vi "Scan_ProFile_CSV_integral.vi"(5 "ProFile Path":path, 7 "Step Size in mm":sgl, 8 "Y-Axis":sgl, 9 "X-Axis":sgl, 10 "Offset Y-Axis":sgl, 11 "Offset X-Axis":sgl) -> ()   [LabVIEW 2016]
uses:
  Utility/Global Constants.vi
panel:
  out "Current Y-Step":i32
  out "Current X-Step":i32
  out "Status?":bool
  out "Abort in Progress":bool
  out "RS":bool
  in  "Abort!":bool
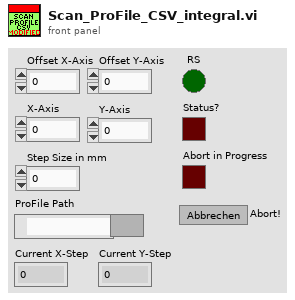
[diagram p1: front panel]
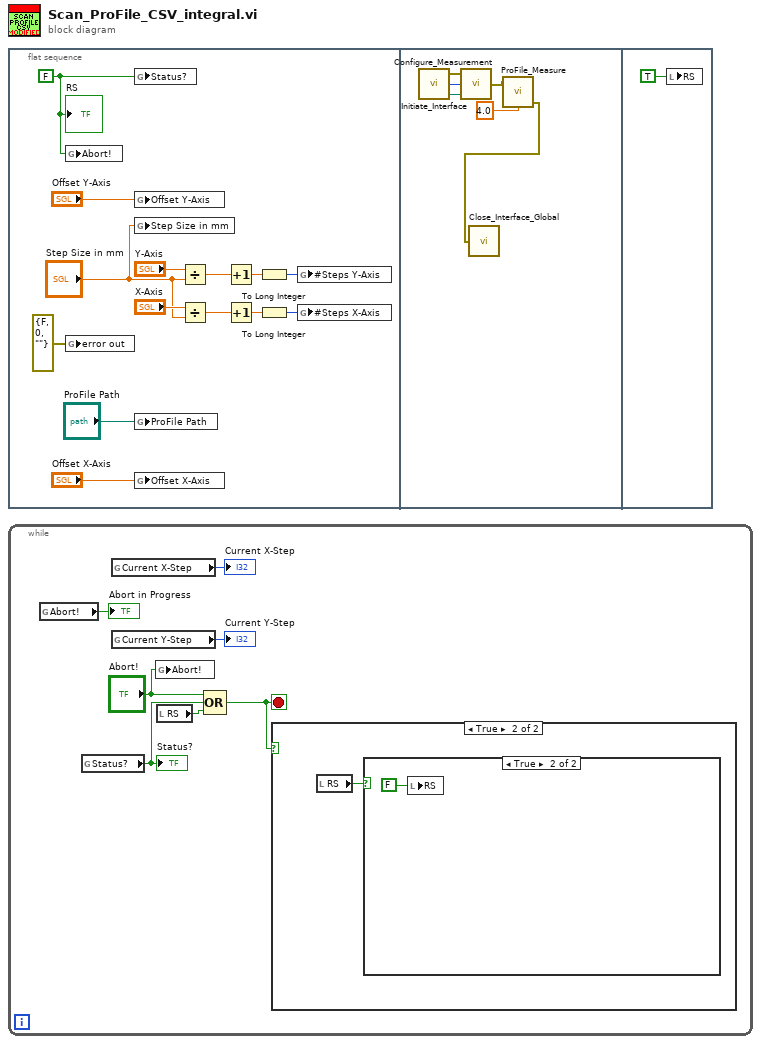
[diagram p0: block diagram]
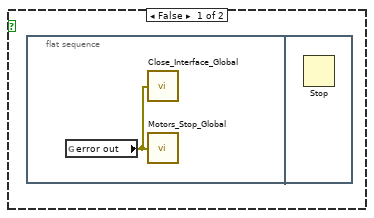
[diagram p3: hidden frame]
diagram:
  n1 = flat-sequence "Flache Sequenzstruktur" {
    frame #0 {
      w2 = FALSE
      n2 = global write "Global Constants.vi" "Abort!"(w2) -> ()
      n3 = global write "Global Constants.vi" "error out"(errorcluster {"status"=FALSE, "code"=0, "source"=""} ("error")) -> ()
      n4 = global write "Global Constants.vi" "Status?"(w2) -> ()
      n5 = global write "Global Constants.vi" "Offset Y-Axis"("Offset Y-Axis") -> ()
      n6 = global write "Global Constants.vi" "Step Size in mm"("Step Size in mm") -> ()
      n7 = global write "Global Constants.vi" "ProFile Path"("ProFile Path") -> ()
      n8 = global write "Global Constants.vi" "Offset X-Axis"("Offset X-Axis") -> ()
      n9 = Divide(x="Y-Axis", y="Step Size in mm") -> (x/y=w12:sgl)
      n10 = Divide(x="X-Axis", y="Step Size in mm") -> (x/y=w11:sgl)
      n11 = Increment(x=w12) -> (x+1=w14:sgl)
      n12 = Increment(x=w11) -> (x+1=w13:sgl)
      n13 = To Long Integer(number=w14) -> (32bit integer=w9:i32)
      n14 = To Long Integer(number=w13) -> (32bit integer=w10:i32)
      n15 = global write "Global Constants.vi" "#Steps Y-Axis"(w9) -> ()
      n16 = global write "Global Constants.vi" "#Steps X-Axis"(w10) -> ()
      "RS" <- w2
    }
    frame #1 {
      n17 = call "Initiate_Interface.vi"() -> ("DLL-Path"=w18:path, "instanceHandle"=w19:u32, "Fehler (Ausgang)"=w20:errorcluster)
      n18 = call "Configure_Measurement.vi"("DLL-Path"=w18, "instanceHandle"=w19, "Error In"=w20) -> ("Fehler (Ausgang)"=w17:errorcluster)
      n19 = call "ProFile_Measure.vi"("Ceiling"=sgl 4.0, "error in"=w17) -> ("error out"=w16:errorcluster)
      n20 = call "Close_Interface_Global.vi"("Error In"=w16) -> ()
    }
    frame #2 {
      n21 = local write "RS"(TRUE) -> ()
    }
  }
  n22 = while {
    stop <- w26 stop-if-true
    n23 = global read "Global Constants.vi" "Abort!"() -> (→"Abort in Progress":bool)
    n24 = global read "Global Constants.vi" "Status?"() -> (w22:bool)
    "Status?" <- w22
    n25 = global read "Global Constants.vi" "Current X-Step"() -> (→"Current X-Step":i32)
    n26 = global read "Global Constants.vi" "Current Y-Step"() -> (→"Current Y-Step":i32)
    n27 = global write "Global Constants.vi" "Abort!"("Abort!") -> ()
    n28 = local read "RS"() -> (w27:bool)
    n29 = Compound Arithmetic op=OR("Abort!", w22, w27) -> (w26:bool)
    n30 = case shown="True" w26 {
      frame False {
      }
      frame True {
        n31 = local read "RS"() -> (w29:bool)
        n32 = case shown="True" w29 {
          frame False {
            n33 = flat-sequence {
              frame #0 {
                n34 = global read "Global Constants.vi" "error out"() -> (w30:errorcluster)
                n35 = call "Close_Interface_Global.vi"("Error In"=w30) -> ()
                n36 = call "Motors_Stop_Global.vi"("error in"=w30) -> ()
              }
              frame #1 {
                n37 = Stop() -> ()  [unwired: 1 in]
              }
            }
          }
          frame True {
            n38 = local write "RS"(FALSE) -> ()
          }
        }
      }
    }
  }
